vi "WfmToSpreadsheet.vi"() -> ()   [LabVIEW 2017]
uses:
  <vilib>/Waveform/WDTFileIO.llb/Read Waveform from File.vi
  <vilib>/Waveform/WDTFileIO.llb/Export Waveforms To Spreadsheet File (1D).vi
panel:
  out "Waveform Chart":waveform(dbl)[](graph)
  out "new file path (Not A Path if cancelled)":path
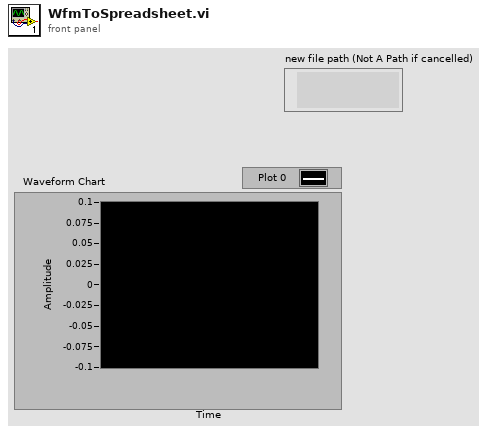
[diagram p1: front panel]
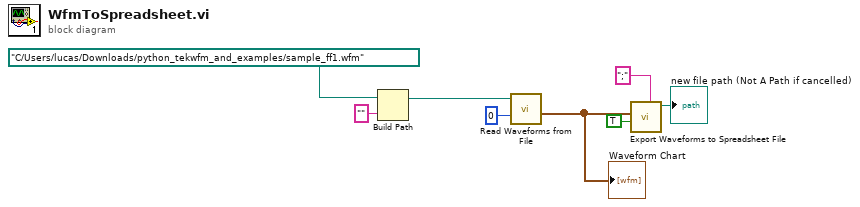
[diagram p0: block diagram]
diagram:
  n1 = Build Path(base path=path "C:/Users/lucas/Downloads/python_tekwfm_and_examples/sample_ff1.wfm" ("file path (dialog if empty)"), name or relative path="") -> (appended path=w7:path)
  n2 = call-poly <vilib>:"Read Waveforms from File.vi"("offset (records:0)"=0, "file path (dialog if empty)"=w7) -> ("all waveforms in record"=w1:waveform(dbl)[])  [unwired: 4 in, 3 out]
  "Waveform Chart" <- w1
  n3 = call-poly <vilib>:"Export Waveforms to Spreadsheet File.vi"("delimiter (Tab)"=";", "multiple time columns? (single:F)"=TRUE, "waveforms"=w1) -> ("new file path (Not A Path if cancelled)"=→"new file path (Not A Path if cancelled)":path)  [unwired: 7 in, 1 out]
